vi "Launch WF progress bar.vi"(10 "Title":string, 11 "Numeric":i32) -> (0 "error out":errorcluster, 3 "ProgressBar_WireFlow out":refnum<class "ProgressBar_WireFlow.lvclass">)   [LabVIEW 2013]
uses:
  <vilib>/addons/WireFlow/_WF_ProgressBar.llb/ProgressBar_WireFlow.lvclass
  <vilib>/addons/WireFlow/_WF_ProgressBar.llb/MessageTextType.ctl
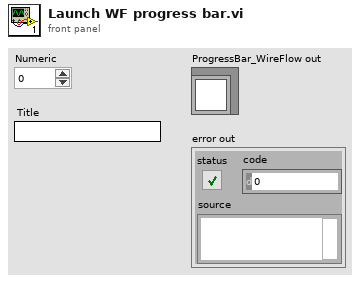
[diagram p1: front panel]
types:
  T1 = typedef "ProgressBar_WireFlow.lvclass/MessageTextType.ctl" = enum16{"Title", "General", "Current item"}
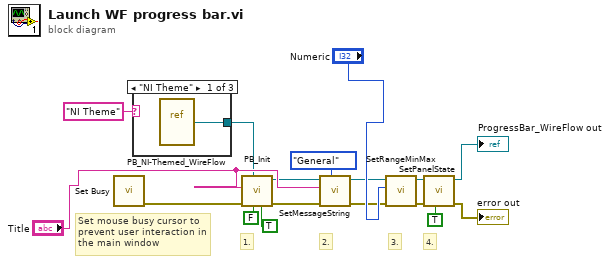
[diagram p0: block diagram]
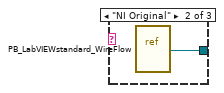
[diagram p2: hidden frame]
diagram:
  # "Set mouse busy cursor to prevent user interaction in the main window"
  # "4."
  # "3."
  # "2."
  # "1."
  n1 = call <vilib>:"Set Busy.vi"() -> ("error out"=w1:errorcluster)  [unwired: 10 in, 1 out]
  n2 = case shown="\"NI Theme\"" "NI Theme" {
    tunnel: [w18 w19 _] -> w8
    frame "NI Theme" {
      n3 = vi-ref "PB_NI-Themed_WireFlow.vi"() -> (w18:refnum<vi>)
    }
    frame "NI Original" {
      n4 = vi-ref "PB_LabVIEWstandard_WireFlow.vi"() -> (w19:refnum<vi>)
    }
    frame Default {
    }
  }
  n5 = call <vilib>:"PB_Init.vi"("Cancel button active? (False)"=TRUE, "Open (TRUE)"=FALSE, "Progress VI"=w8, "error in (no error)"=w1, "title (\"Progress\")"="Title") -> ("error out"=w4:errorcluster, "WF-ProgressBar out"=w6:refnum<class "ProgressBar_WireFlow.lvclass">)  [unwired: 5 in]
  n6 = call-dynamic "SetMessageString.vi"("message field"=MessageTextType."General", "error in (no error)"=w4, "Message"="Title", "WF-ProgressBar in"=w6) -> ("error out"=w3:errorcluster, "WF-ProgressBar out"=w5:refnum<class "ProgressBar_WireFlow.lvclass">)  [unwired: 6 in]
  n7 = call-dynamic "SetRangeMinMax.vi"("error in (no error)"=w3, "Max (1)"="Numeric", "WF-ProgressBar in"=w5) -> ("error out"=w10:errorcluster, "WF-ProgressBar out"=w11:refnum<class "ProgressBar_WireFlow.lvclass">)  [unwired: 7 in]
  n8 = call-dynamic "SetPanelState.vi"("State (T = Open)"=TRUE, "error in (no error)"=w10, "WF-ProgressBar in"=w11) -> ("error out"=→"error out":errorcluster, "WF-ProgressBar out"=→"ProgressBar_WireFlow out":refnum<class "ProgressBar_WireFlow.lvclass">)  [unwired: 7 in]
